vi "Controller - Select Message.vi"(8 "error in (no error)":errorcluster, 10 "Message Name":T1, 11 "Messages":string[](array[string])) -> (0 "error out":errorcluster, 3 "Message":string)   [LabVIEW 2017]
doc: "Reads all messages of ATM controllerfrom external file."
uses:
  Controls/Controller Message Name.ctl
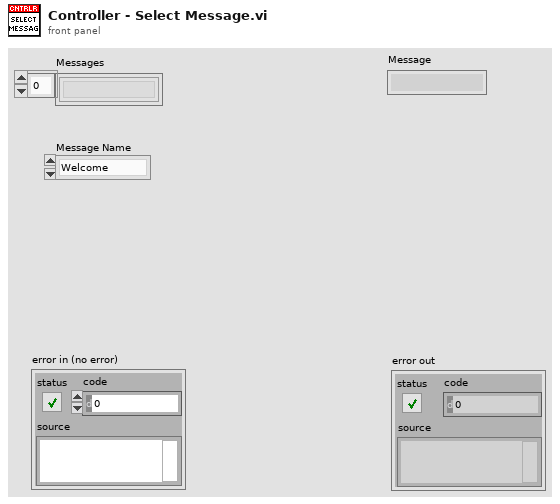
[diagram p1: front panel]
types:
  T1 = typedef "Controller Message Name.ctl" = enum16{"Welcome", "Login", "Idle", "Invalid Login", "Terminate", "Deposit", "Withdrawal", "Fast Cash", "Withdrawal Complete", "Withdrawal Failed", "Balance Inquiry"}
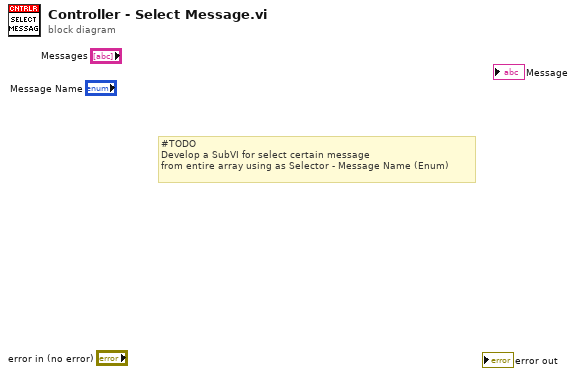
[diagram p0: block diagram]
diagram:
  # "#TODO\nDevelop a SubVI for select certain message\nfrom entire array using as Selector - Message Name (Enum)"
